vi "PKG_IMC_GetEncp.vi"(9 "axisnum":i32, 10 "pos":i32[](array[numeric])=array[4097 elements], 11 "Handle":u32) -> (1 "function return":i32, 2 "pos out":i32[](array[numeric]), 3 "Handle out":u32)   [LabVIEW 2018, in "IMC_Pkg4xxx.lvlib"]
doc: "PKG_IMC_GetEncp(IMC_HANDLE Handle, long pos[], int axisnum);"
uses:
  IMC_Pkg4xxx.lvlib
  IMC_Pkg4xxx.dll
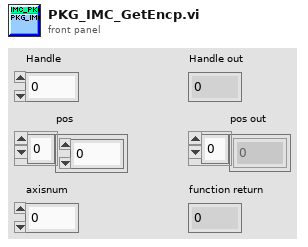
[diagram p1: front panel]
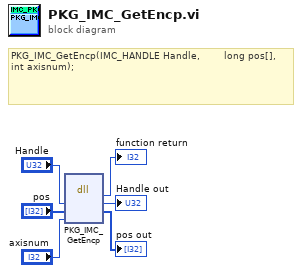
[diagram p0: block diagram]
diagram:
  # "PKG_IMC_GetEncp(IMC_HANDLE Handle, \t\t \t\t\t\tlong pos[], \t\t\t\t\t\t\t\tint axisnum);"
  n1 = dll-call lib="PTH2\\abs D做的项目航天测量驱动电机IMCAppincLabview32\nIMC_Pkg4xxx.*" fn="PKG_IMC_GetEncp"("Handle"="Handle", "pos"="pos", "axisnum"="axisnum") -> (→"function return":i32, "Handle"=→"Handle out":u32, "pos"=→"pos out":i32[])  [unwired: 4 in, 2 out]
